vi "DB Execute Special Query.vi"(7 "table Name":string, 8 "error in (no error)":errorcluster, 11 "Db Reference":refnum<k24>) -> (0 "error out":errorcluster, 2 "Data":string[][](array[string]), 3 "Db Reference":refnum<k24>)   [LabVIEW 2020]
uses:
  D:/Labview/Auto Run Screen/Source Code/Database/Support/dbquery.dll
  Support/dbquery.dll
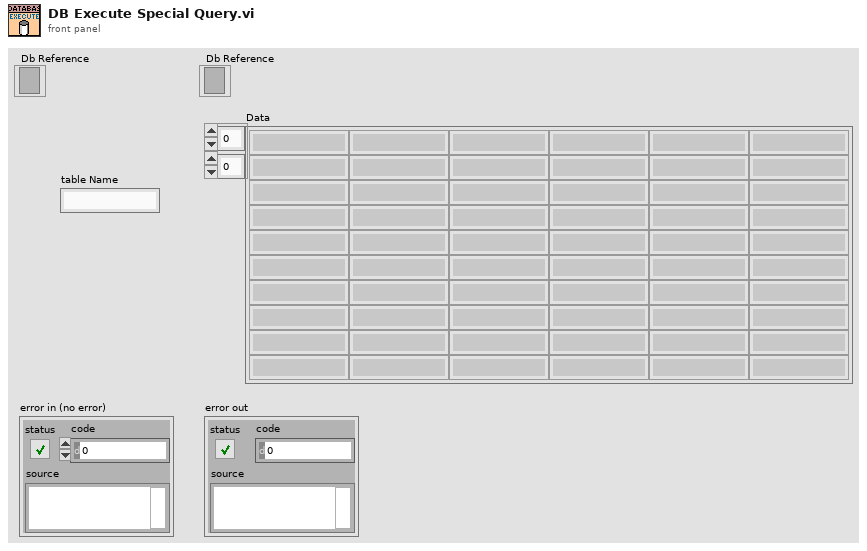
[diagram p1: front panel]
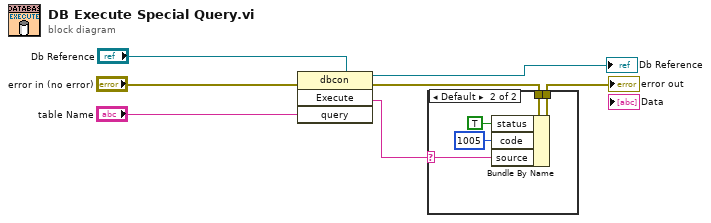
[diagram p0: block diagram]
diagram:
  n1 = invoke class="dbcon" method="Execute"(reference="Db Reference", error in="error in (no error)", "query"="table Name") -> (reference out=→"Db Reference":refnum<k24>, error out=w4:errorcluster, "Execute"=w1:string)  [unwired: 1 in, 1 out]
  n2 = case shown="Default" w1 {
    selector: w1 -> [_ w10]
    tunnel: w4 -> [w8 w13]
    tunnel: [w8 w12] -> w2
    frame "" {
    }
    frame Default {
      n3 = Bundle By Name(cluster=w13, "status"=TRUE, "code"=1005, "source"=w10) -> (w12:errorcluster)
    }
  }
  "error out" <- w2
